vi "Untitled 2.vi"() -> ()   [LabVIEW 2014]
uses:
  <instrlib>/niUSRP/niUSRP Write Tx Data (CDB).vi
panel:
  in  "device name":refnum<k15>="192.168.10.2"
  out "Error Out":errorcluster
  in  "active antenna":string="TX/RX"
  in  "Stop Button":bool
  out "Waveform Graph":dbl[](graph)
  out "IQ Plot":dbl[](graph)
  out "Gain [dB] (actual)":dbl format="%#.6p"
  out "Carrier Frequency \n[Hz] (actual)":dbl=2450000000.0 format="%#.6p"
  out "IQ Sampling\nRate [s/sec] (actual)":dbl=10000000.0 format="%#.6p"
  in  "Gain [dB]":dbl format="%#.6p"
  in  "Carrier\nFrequency [Hz]":dbl=915000000.0 format="%#.6p"
  in  "IQ Sampling\nRate [s/sec]":dbl=10000000.0 format="%#.6p"
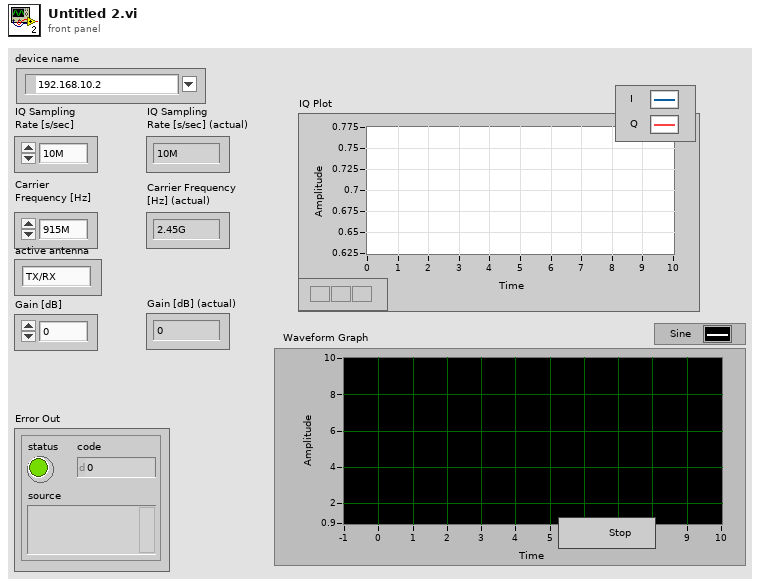
[diagram p1: front panel]
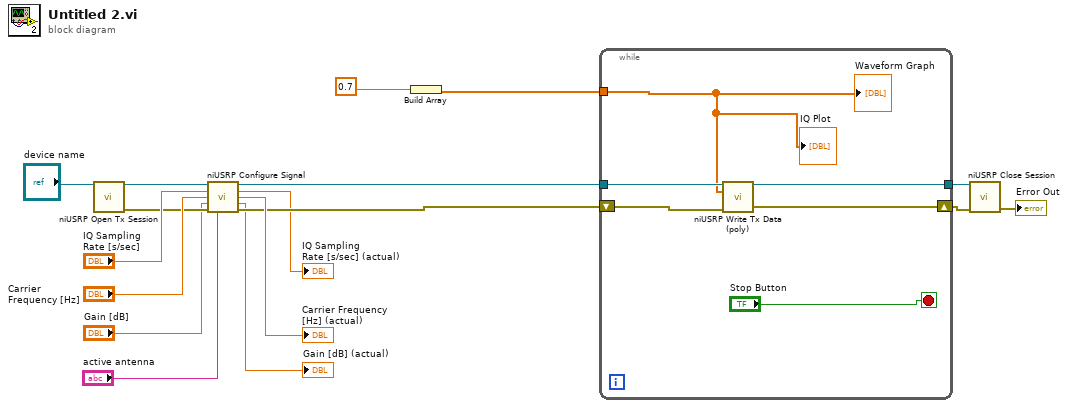
[diagram p0: block diagram]
diagram:
  n1 = call <instrlib>:"niUSRP Open Tx Session.vi"("device names"="device name") -> ("session handle out"=w17:refnum<k15>, "error out"=w14:errorcluster)  [unwired: 13 in]
  n2 = call <instrlib>:"niUSRP Configure Signal.vi"("session handle"=w17, "IQ rate"="IQ Sampling\nRate [s/sec]", "carrier frequency"="Carrier\nFrequency [Hz]", "gain"="Gain [dB]", "error in (no error)"=w14, "active antenna"="active antenna") -> ("session handle out"=w12:refnum<k15>, "coerced IQ rate"=→"IQ Sampling\nRate [s/sec] (actual)":dbl, "coerced carrier frequency"=→"Carrier Frequency \n[Hz] (actual)":dbl, "coerced gain"=→"Gain [dB] (actual)":dbl, "error out"=w11:errorcluster)  [unwired: 5 in]
  n3 = Build Array(0.7) -> (w1:dbl[])
  n4 = while {
    tunnel: w12 -> [w23]
    tunnel: [w21] -> w10
    tunnel: w1 -> [w19]
    shift-right: [w18] -> w3
    shift-left: w11 -> [w22]
    stop <- "Stop Button" stop-if-true
    n5 = call-poly <instrlib>:"niUSRP Write Tx Data (poly).vi"("session handle"=w23, "data"=w19, "error in (no error)"=w22) -> ("session handle out"=w21:refnum<k15>, "error out"=w18:errorcluster)  [unwired: 11 in]
    "Waveform Graph" <- w19
    "IQ Plot" <- w19
  }
  n6 = call <instrlib>:"niUSRP Close Session.vi"("session handle"=w10, "error in (no error)"=w3) -> ("error out"=→"Error Out":errorcluster)  [unwired: 13 in]
